vi "Deposit.vi"(8 "error in (no error)":errorcluster, 10 "Amount":dbl, 11 "ACreditAccount in":refnum<class "ACreditAccount.lvclass">) -> (0 "error out":errorcluster, 2 "Balance":dbl, 3 "ACreditAccount out":refnum<class "ACreditAccount.lvclass">)   [LabVIEW 2020, in "ACreditAccount.lvclass"]
uses:
  ACreditAccount.lvclass
  ACreditAccount.lvclass/ACreditAccount.ctl
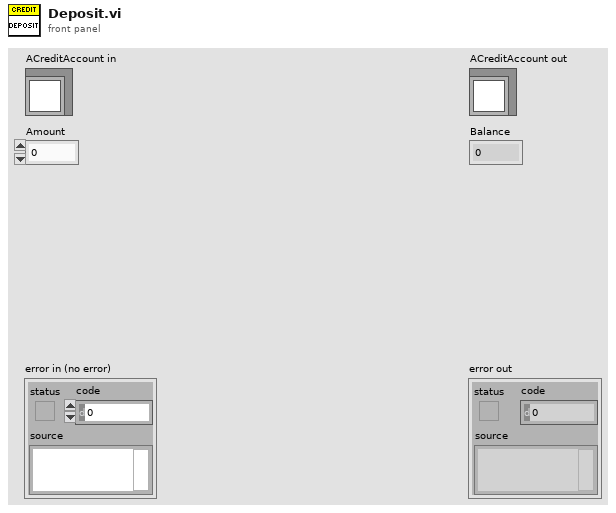
[diagram p1: front panel]
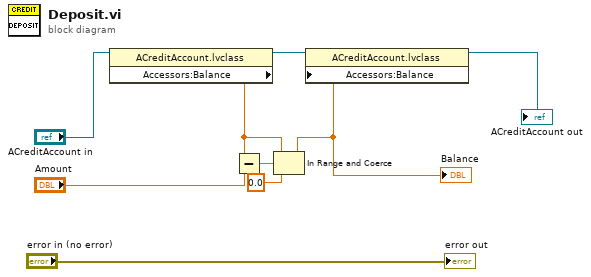
[diagram p0: block diagram]
diagram:
  n1 = property class="ACreditAccount.lvclass"(reference="ACreditAccount in") -> (reference out=w3:refnum<class "ACreditAccount.lvclass">, "Accessors:Balance"=w4:dbl)  [unwired: 1 in, 1 out]
  n2 = Subtract(x=w4, y="Amount") -> (x-y=w6:dbl)
  n3 = In Range and Coerce(upper limit=w4, x=w6, lower limit=0.0) -> (coerced(x)=w1:dbl)  [unwired: 1 out]
  "Balance" <- w1
  n4 = property class="ACreditAccount.lvclass"(reference=w3, "Accessors:Balance"=w1) -> (reference out=→"ACreditAccount out":refnum<class "ACreditAccount.lvclass">)  [unwired: 1 in, 1 out]
  "error out" <- "error in (no error)"
